vi "onHttpPatch (Buffer).vi"(6 "timeout":i32=10000, 7 "output file":path, 8 "error in":errorcluster, 9 "buffer":string, 10 "url":string, 11 "advanced-http-client in":refnum<class "advanced-http-client.lvclass">) -> (0 "error out":errorcluster, 1 "body":string, 2 "headers":string, 3 "advanced-http-client out":refnum<class "advanced-http-client.lvclass">)   [LabVIEW 2020, in "REST Client.lvlib" / "advanced-http-client.lvclass"]
uses:
  advanced-http-client.lvclass
  advanced-http-client.lvclass/advanced-http-client.ctl
  <vilib>/NI/Advanced HTTP Client/PATCH (Buffer).vi
  <vilib>/NI/Advanced HTTP Client/Session.lvclass
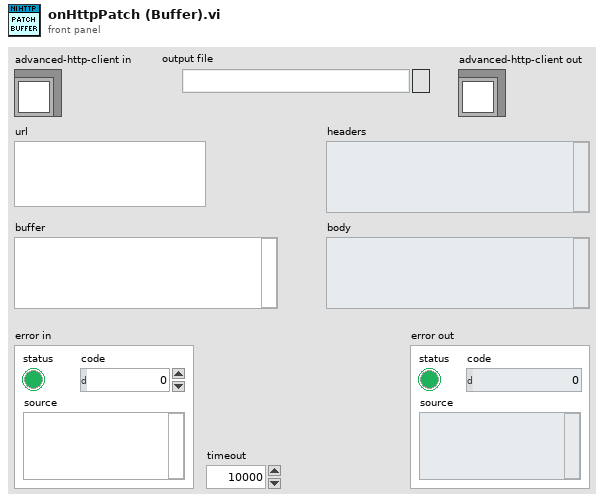
[diagram p1: front panel]
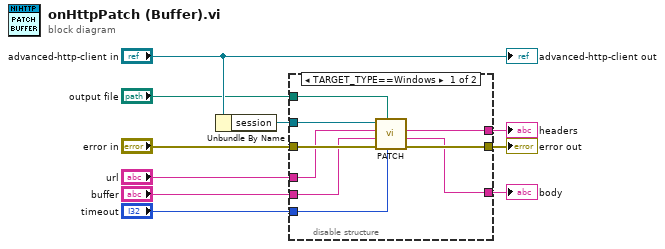
[diagram p0: block diagram]
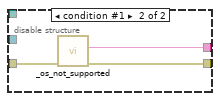
[diagram p2: hidden frame]
diagram:
  n1 = Unbundle By Name("advanced-http-client in") -> ("session"=w9:refnum<class "Session.lvclass">)
  n2 = disable-structure shown="TARGET_TYPE==Windows" {
    disable-tunnel: w9 -> [w19 _]
    disable-tunnel: "error in" -> [w18 w22]
    disable-tunnel: [w17 w21] -> w7
    disable-tunnel: "buffer" -> [w16 _]
    disable-tunnel: "url" -> [w15 _]
    disable-tunnel: "output file" -> [w14 _]
    disable-tunnel: "timeout" -> [w13 _]
    disable-tunnel: [w12 w20] -> w2
    disable-tunnel: [w11 _] -> w1
    frame condition #0 (active) {
      n3 = call-poly <vilib>:"PATCH.vi"("timeout"=w13, "output file"=w14, "error in"=w18, "buffer"=w16, "url"=w15, "session in"=w19) -> ("error out"=w17:errorcluster, "body"=w11:string, "headers"=w12:string)  [unwired: 1 in, 2 out]
    }
    frame condition #1 {
      n4 = call "_os_not_supported.vi"("error in (no error)"=w22) -> ("error out"=w21:errorcluster, "headers"=w20:string)  [unwired: 9 in]
    }
  }
  "error out" <- w7
  "headers" <- w2
  "body" <- w1
  "advanced-http-client out" <- "advanced-http-client in"
